vi "WiiMote Read IR.vi"(2 "error in":errorcluster, 3 "IRState":refnum<k24>) -> (0 "error out":errorcluster, 1 "IRState":T1 {"Mode" items=["Off"=0, "Basic"=1, "Extended"=3, "Full"=5]})   [LabVIEW 2011]
uses:
  D:/jjensen/Documents/Lab Book/embeddedLab/exercises/LabVIEW/.WiiMote/Dependencies/WiimoteLib.dll
  .WiiMote/Dependencies/WiimoteLib.dll
  WiiMote State with IR.ctl
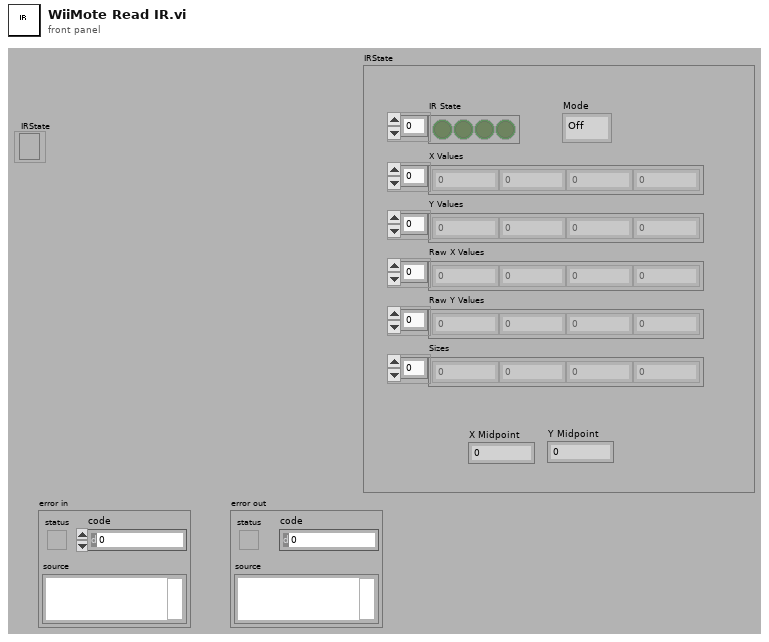
[diagram p1: front panel]
types:
  T1 = typedef "WiiMote State with IR.ctl" = cluster{"Mode":u8, "IR State":bool[], "X Values":sgl[], "Y Values":sgl[], "Raw X Values":i32[], "Raw Y Values":i32[], "Sizes":i32[], "X Midpoint":sgl, "Y Midpoint":sgl}
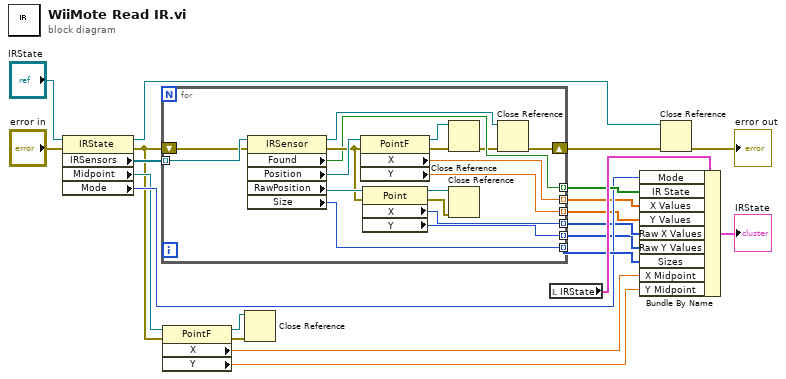
[diagram p0: block diagram]
diagram:
  n1 = property class="IRState"(reference="IRState", error in="error in") -> (reference out=w1:refnum<k24>, error out=w8:errorcluster, "IRSensors"=w17:refnum<k24>[], "Midpoint"=w9:refnum<k24>, "Mode"=w14:u8)
  n2 = for {
    tunnel: w17 -> [w39] mode=indexing
    shift-right: [w22] -> w3
    shift-left: w8 -> [w38]
    tunnel: [w34] -> w16 mode=indexing
    tunnel: [w33] -> w15 mode=indexing
    tunnel: [w32] -> w13 mode=indexing
    tunnel: [w31] -> w12 mode=indexing
    tunnel: [w30] -> w11 mode=indexing
    tunnel: [w29] -> w10 mode=indexing
    n3 = property class="IRSensor"(reference=w39, error in=w38) -> (reference out=w23:refnum<k24>, error out=w35:errorcluster, "Found"=w33:bool, "Position"=w37:refnum<k24>, "RawPosition"=w36:refnum<k24>, "Size"=w34:i32)
    n4 = property class="PointF"(reference=w37, error in=w35) -> (reference out=w26:refnum<k24>, error out=w25:errorcluster, "X"=w32:sgl, "Y"=w31:sgl)
    n5 = property class="Point"(reference=w36, error in=w35) -> (reference out=w27:refnum<k24>, error out=w28:errorcluster, "X"=w30:i32, "Y"=w29:i32)
    n6 = Close Reference(reference=w26, error in (no error)=w25) -> (error out=w24:errorcluster)
    n7 = Close Reference(reference=w27, error in (no error)=w28) -> ()  [unwired: 1 out]
    n8 = Close Reference(reference=w23, error in (no error)=w24) -> (error out=w22:errorcluster)
  }
  n9 = property class="PointF"(reference=w9, error in=w8) -> (reference out=w4:refnum<k24>, error out=w5:errorcluster, "X"=w7:sgl, "Y"=w6:sgl)
  n10 = Close Reference(reference=w4, error in (no error)=w5) -> ()  [unwired: 1 out]
  n11 = local read "IRState"() -> (w19:T1)
  n12 = Bundle By Name(cluster=w19, "Mode"=w14, "IR State"=w15, "X Values"=w13, "Y Values"=w12, "Raw X Values"=w11, "Raw Y Values"=w10, "Sizes"=w16, "X Midpoint"=w7, "Y Midpoint"=w6) -> (→"IRState":T1)
  n13 = Close Reference(reference=w1, error in (no error)=w3) -> (error out=→"error out":errorcluster)
